vi "Comm_Read.vi"(4 "Params":cluster{"bytes":i32, "timeout (ms)":i32}={"bytes"=1, "timeout (ms)"=100}, 6 "Task":enum16{"Instant", "All", "AllFast", "Params"}(ring), 8 "error in (no error)":errorcluster, 11 "Python":T1) -> (0 "error out":errorcluster, 1 "Text read":string)   [LabVIEW 2022 SP3]
uses:
  PythonCtrl.ctl
  Processors.ctl
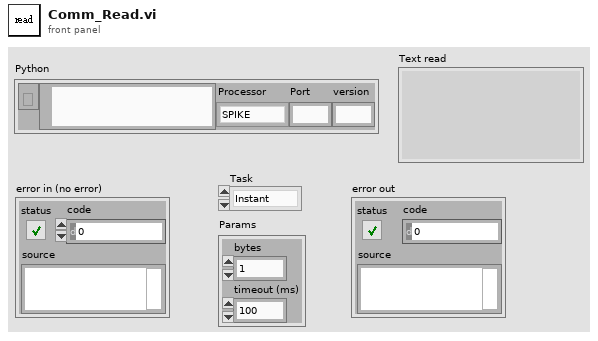
[diagram p1: front panel]
types:
  T1 = typedef "PythonCtrl.ctl" = cluster{"session":refnum<k35>, "PyPath":path, "Processor":T2, "Port":string, "version":string}
  T2 = typedef "Processors.ctl" = enum16{"SPIKE", "Pi", "Pi_ssh", "OpenMV", "Dunio"}
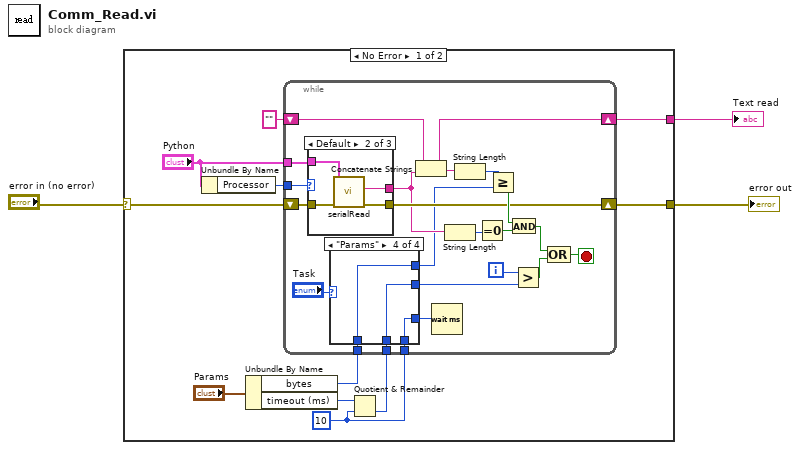
[diagram p0: block diagram]
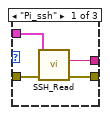
[diagram p2: hidden frame]
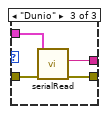
[diagram p3: hidden frame]
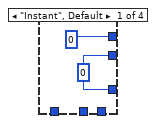
[diagram p4: hidden frame]
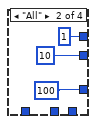
[diagram p5: hidden frame]
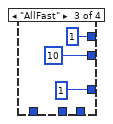
[diagram p6: hidden frame]
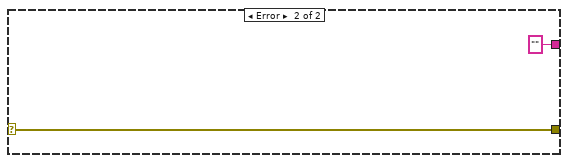
[diagram p7: hidden frame]
diagram:
  n1 = case shown="No Error" "error in (no error)" {
    selector: "error in (no error)" -> [w4 w61]
    tunnel: [w14 w61] -> w3
    tunnel: [w12 ""] -> w2
    frame No Error {
      w6 = u32 10 ("y")
      n2 = Unbundle By Name("Python") -> ("Processor"=w10:T2)
      n3 = Unbundle By Name("Params") -> ("bytes"=w8:i32, "timeout (ms)"=w7:i32)
      n4 = Quotient & Remainder(x=w7, y=w6) -> (floor(x/y)=w5:u32)  [unwired: 1 out]
      n5 = while {
        shift-right: [w24] -> w14
        shift-left: w4 -> [w25]
        shift-right: [w34] -> w12
        shift-left: "" -> [w36]
        tunnel: "Python" -> [w22]
        tunnel: w10 -> [w20]
        tunnel: w8 -> [w17]
        tunnel: w6 -> [w16]
        tunnel: w5 -> [w15]
        i -> [w29]
        stop <- w31 stop-if-true
        n6 = case shown="Default" w20 {
          tunnel: w25 -> [w39 w44 w48]
          tunnel: [w38 w43 w47] -> w24
          tunnel: w22 -> [w40 w42 w46]
          tunnel: [w37 w41 w45] -> w21
          frame "Pi_ssh" {
            n7 = call "SSH_Read.vi"("error in (no error)"=w39, "Python"=w40) -> ("error out"=w38:errorcluster, "Reply"=w37:string)  [unwired: 7 in, 1 out]
          }
          frame Default {
            n8 = call "serialRead.vi"("error in (no error)"=w44, "Python"=w42) -> ("error out"=w43:errorcluster, "Reply"=w41:string)  [unwired: 7 in, 1 out]
          }
          frame "Dunio" {
            n9 = call "serialRead.vi"("error in (no error)"=w48, "Python"=w46) -> ("error out"=w47:errorcluster, "Reply"=w45:string)  [unwired: 7 in, 1 out]
          }
        }
        n10 = case shown="\"Params\"" "Task" {
          tunnel: [w50 10 ("y") 10 ("y") w57] -> w28
          tunnel: [w50 u32 100 ("milliseconds to wait") u32 1 ("milliseconds to wait") w58] -> w26
          tunnel: [0 ("y") 1 ("y") 1 ("y") w59] -> w18
          tunnel: w17 -> [_ _ _ w59]
          tunnel: w16 -> [_ _ _ w58]
          tunnel: w15 -> [_ _ _ w57]
          frame "Instant", Default {
            w50 = u32 0 ("y")
          }
          frame "All" {
          }
          frame "AllFast" {
          }
          frame "Params" {
          }
        }
        n11 = Concatenate Strings(w36, w21) -> (w34:string)
        n12 = Wait (ms)(milliseconds to wait=w26) -> ()  [unwired: 1 out]
        n13 = String Length(string=w21) -> (length=w35:i32)
        n14 = String Length(string=w34) -> (length=w19:i32)
        n15 = Equal To 0?(x=w35) -> (x = 0?=w32:bool)
        n16 = Greater Or Equal?(x=w19, y=w18) -> (x >= y?=w33:bool)
        n17 = And(x=w33, y=w32) -> (x .and. y?=w30:bool)
        n18 = Greater?(x=w29, y=w28) -> (0:w27:bool)
        n19 = Compound Arithmetic op=OR(w30, w27) -> (w31:bool)
      }
    }
    frame Error {
    }
  }
  "error out" <- w3
  "Text read" <- w2
